vi "2.4.vi"() -> ()   [LabVIEW 2017]
panel:
  out "Numeric":dbl
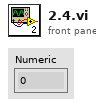
[diagram p1: front panel]
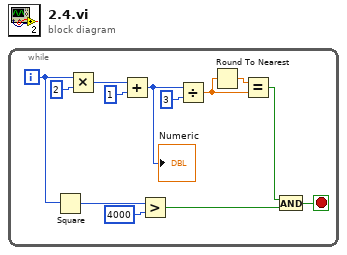
[diagram p0: block diagram]
diagram:
  n1 = while {
    i -> [w1]
    stop <- w4 stop-if-true
    n2 = Square(x=w1) -> (x^2=w8:i32)
    n3 = Multiply(x=w1, y=2) -> (x*y=w13:i32)
    n4 = Add(x=w13, y=1) -> (x+y=w11:i32)
    "Numeric" <- w11
    n5 = Greater?(x=w8, y=4000) -> (0:w3:bool)
    n6 = Divide(x=w11, y=3) -> (x/y=w5:dbl)
    n7 = Round To Nearest(number=w5) -> (nearest integer value=w6:dbl)
    n8 = Equal?(x=w6, y=w5) -> (x = y?=w2:bool)
    n9 = And(x=w2, y=w3) -> (x .and. y?=w4:bool)
  }
